vi "FF+FB 適應性控制(系統鑑別).vi"() -> ()   [LabVIEW 2010]
uses:
  <vilib>/DAQmx/read.llb/DAQmx Read (Analog 1D DBL NChan 1Samp).vi
  <vilib>/DAQmx/write.llb/DAQmx Write (Analog DBL 1Chan 1Samp).vi
  <vilib>/DAQmx/create/channels.llb/DAQmx Create Channel (AI-Voltage-Basic).vi
  <vilib>/DAQmx/configure/timing.llb/DAQmx Timing (Sample Clock).vi
  <vilib>/DAQmx/create/channels.llb/DAQmx Create Channel (AO-Voltage-Basic).vi
  <vilib>/daqmx/miscellaneous.llb/DAQmx Fill In Error Info.vi
panel:
  in  "input channels 3":tag="PXI-6229/ai2"
  in  "適應性雜訊消除":bool=TRUE
  in  "u(收斂係數)":dbl=0.02
  in  "order":i32=1000
  in  "ch2-1估測DC時間(秒)":dbl=2.0
  in  "ch2-2 估測DC時間(秒)":dbl=2.0
  in  "ch2 Kii 增益":dbl
  in  "ch2 Kp 增益":dbl=0.13
  out "overload":bool=TRUE
  in  "ch1 Kp 增益":dbl=-23.0
  in  "ch2 Ki 增益":dbl=83.5
  in  "ch1 Ki 增益":dbl=-600.0
  in  "ch1-2估測DC時間(秒)":dbl=2.0
  in  "ch2-3估測DC時間(秒)":dbl=0.1
  in  "Controller on":bool
  out "error out":errorcluster
  out "延遲百分比(%)  需小於0.5%":dbl=0.21369830071382712
  out "理想迴圈時間(ms)":dbl=0.2
  out "迴圈平均運行時間(ms)":dbl=0.20042739660142767
  in  "output channels 1":tag="PXI-6733/ao0"
  in  "stop":bool
  in  "ch1-1估測DC時間(秒)":dbl=2.0
  in  "每通道取樣頻率(Hz)":dbl=5000.0 format="%0.2f"
  in  "input channels 2":tag="PXI-6229/ai1"
  in  "input channels 1":tag="PXI-6229/ai0"
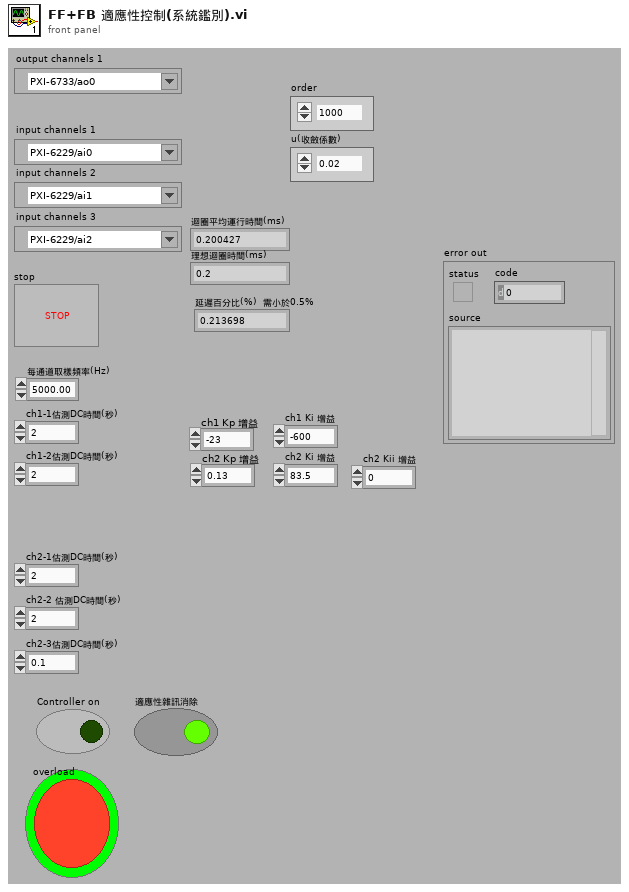
[diagram p1: front panel]
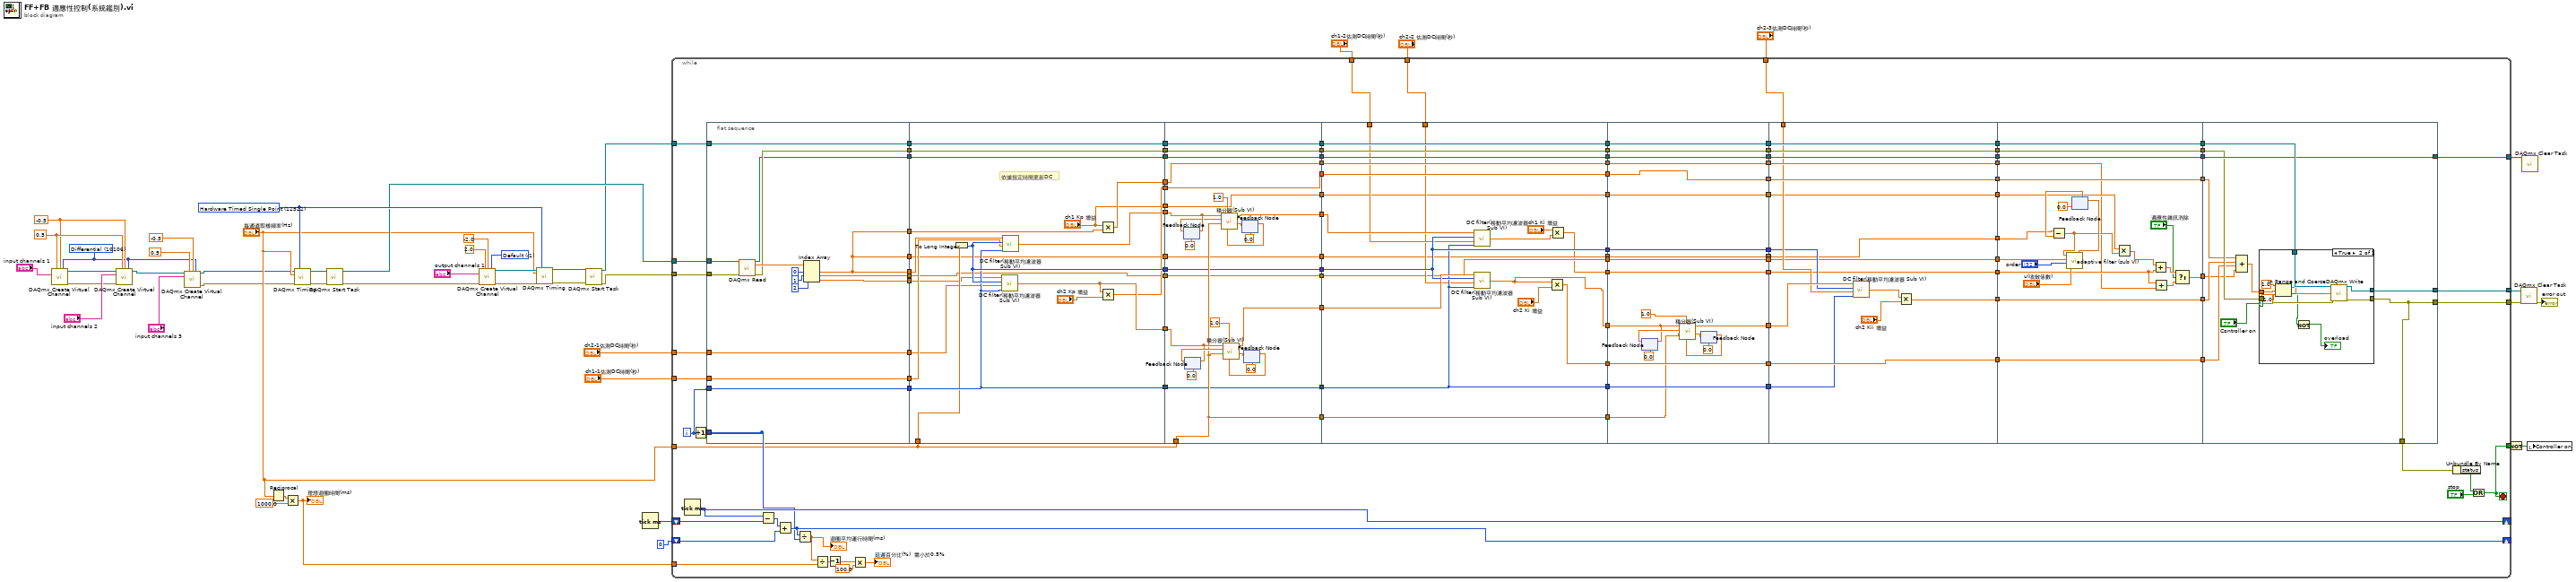
[diagram p0: block diagram]
diagram:
  w35 = -1 items=["Default"=-1, "RSE"=10083, "Differential"=10106, "Pseudodifferential"=12529] ("output terminal configuration")
  w32 = 12522 items=["Finite Samples"=10178, "Continuous Samples"=10123, "Hardware Timed Single Point"=12522] ("sample mode")
  w1 = 10106 items=["default"=-1, "RSE"=10083, "NRSE"=10078, "Differential"=10106, "Pseudodifferential"=12529] ("input terminal configuration")
  w41 = -0.5 ("minimum value")
  w42 = 0.5 ("maximum value")
  n1 = call-poly <vilib>:"DAQmx Create Virtual Channel.vi"("maximum value"=w42, "minimum value"=w41, "input terminal configuration"=w1, "physical channels"="input channels 1") -> ("task out"=w45:refnum<k21>, "error out"=w39:errorcluster)  [unwired: 10 in]
  n2 = call-poly <vilib>:"DAQmx Create Virtual Channel.vi"("task in"=w45, "maximum value"=w42, "minimum value"=w41, "input terminal configuration"=w1, "physical channels"="input channels 2", "error in"=w39) -> ("task out"=w7:refnum<k21>)  [unwired: 8 in, 1 out]
  n3 = call-poly <vilib>:"DAQmx Create Virtual Channel.vi"("task in"=w7, "maximum value"=0.5, "minimum value"=-0.5, "input terminal configuration"=w1, "physical channels"="input channels 3") -> ("task out"=w6:refnum<k21>, "error out"=w5:errorcluster)  [unwired: 9 in]
  n4 = Reciprocal(x="每通道取樣頻率(Hz)") -> (1/x=w23:dbl)
  n5 = Multiply(x=w23, y=1000.0) -> (x*y=w21:dbl)
  "理想迴圈時間(ms)" <- w21
  n6 = call-poly <vilib>:"DAQmx Timing.vi"("task/channels in"=w6, "sample mode"=w32, "rate"="每通道取樣頻率(Hz)", "error in"=w5) -> ("task out"=w40:refnum<k21>, "error out"=w38:errorcluster)  [unwired: 10 in]
  n7 = call <vilib>:"DAQmx Start Task.vi"("task/channels in"=w40, "error in"=w38) -> ("task out"=w28:refnum<k21>, "error out"=w29:errorcluster)  [unwired: 12 in]
  n8 = call-poly <vilib>:"DAQmx Create Virtual Channel.vi"("maximum value"=2.0, "minimum value"=-2.0 ("maximum value"), "output terminal configuration"=w35, "physical channels"="output channels 1", "error in"=w29) -> ("task out"=w34:refnum<k21>, "error out"=w33:errorcluster)  [unwired: 9 in]
  n9 = call-poly <vilib>:"DAQmx Timing.vi"("task/channels in"=w34, "sample mode"=w32, "rate"="每通道取樣頻率(Hz)", "error in"=w33) -> ("task out"=w31:refnum<k21>, "error out"=w30:errorcluster)  [unwired: 10 in]
  n10 = call <vilib>:"DAQmx Start Task.vi"("task/channels in"=w31, "error in"=w30) -> ("task out"=w19:refnum<k21>, "error out"=w27:errorcluster)  [unwired: 12 in]
  n11 = Tick Count (ms)() -> (millisecond timer value=w25:u32)
  n12 = while {
    tunnel: w28 -> [w155]
    tunnel: w27 -> [w154]
    shift-right: [w151] -> _
    shift-left: w25 -> [w152]
    shift-right: [w148] -> _
    shift-left: 0 ("index") -> [w149]
    tunnel: w21 -> [w145]
    tunnel: "每通道取樣頻率(Hz)" -> [w102]
    tunnel: w19 -> [w132]
    tunnel: [w126] -> w16
    tunnel: [w100] -> w15
    tunnel: [w115] -> w14
    tunnel: "ch1-1估測DC時間(秒)" -> [w114]
    tunnel: [w101] -> w12
    tunnel: "ch1-2估測DC時間(秒)" -> [w86]
    tunnel: "ch2-3估測DC時間(秒)" -> [w85]
    tunnel: "ch2-2 估測DC時間(秒)" -> [w84]
    tunnel: "ch2-1估測DC時間(秒)" -> [w83]
    i -> [w112]
    stop <- w101 stop-if-true
    n13 = Tick Count (ms)() -> (millisecond timer value=w151:u32)
    n14 = Increment(x=w112) -> (x+1=w147:i32)
    n15 = flat-sequence {
      tunnel: w155 -> [w170]
      tunnel: w154 -> [w169]
      tunnel: [w158] -> w153
      tunnel: w147 -> [_]
      tunnel: w132 -> [w165]
      tunnel: [w165] -> w127
      tunnel: [w164] -> w125
      tunnel: [w163] -> w120
      tunnel: w114 -> [w162]
      tunnel: [w162] -> w113
      tunnel: w112 -> [w161]
      tunnel: [w161] -> w111
      tunnel: w83 -> [w160]
      tunnel: [w160] -> w82
      tunnel: [w158] -> w63
      tunnel: [w159] -> w62
      tunnel: [w158] -> w53
      tunnel: [w156] -> w46
      tunnel: w153 -> [w186]
      tunnel: [w179] -> w140
      tunnel: [w176] -> w139
      tunnel: [w189] -> w128
      tunnel: w127 -> [w189]
      tunnel: w125 -> [w188]
      tunnel: [w188] -> w124
      tunnel: w120 -> [w187]
      tunnel: [w187] -> w116
      tunnel: w113 -> [w184]
      tunnel: w111 -> [w183]
      tunnel: [w185] -> w109
      tunnel: [w183] -> w107
      tunnel: w102 -> [w182]
      tunnel: [w181] -> w95
      tunnel: [w178] -> w91
      tunnel: w82 -> [w177]
      tunnel: [w175] -> w64
      tunnel: w63 -> [w175]
      tunnel: w62 -> [w174]
      tunnel: [w174] -> w61
      tunnel: w53 -> [w173]
      tunnel: ["ch1 Kp 增益"] -> w48
      tunnel: w46 -> [w171]
      tunnel: w140 -> [w205]
      tunnel: w139 -> [w216]
      tunnel: w102 -> [w202]
      tunnel: [w204] -> w138
      tunnel: [w203] -> w137
      tunnel: [w202] -> w134
      tunnel: [w201] -> w129
      tunnel: w128 -> [w201]
      tunnel: w124 -> [w200]
      tunnel: [w200] -> w122
      tunnel: [w199] -> w117
      tunnel: w116 -> [w199]
      tunnel: [w198] -> w110
      tunnel: w109 -> [w198]
      tunnel: [w197] -> w108
      tunnel: w107 -> [w197]
      tunnel: w95 -> [w194]
      tunnel: [w194] -> w92
      tunnel: w91 -> [w193]
      tunnel: [w193] -> w90
      tunnel: [w192] -> w65
      tunnel: w64 -> [w192]
      tunnel: w61 -> [w191]
      tunnel: [w191] -> w60
      tunnel: [w190] -> w49
      tunnel: w48 -> [w190]
      tunnel: w138 -> [w233]
      tunnel: w137 -> [w232]
      tunnel: [w225] -> w136
      tunnel: [w237] -> w135
      tunnel: w134 -> [w237]
      tunnel: [w236] -> w130
      tunnel: w129 -> [w236]
      tunnel: [w235] -> w123
      tunnel: w122 -> [w235]
      tunnel: [w234] -> w118
      tunnel: w117 -> [w234]
      tunnel: w110 -> [w231]
      tunnel: w108 -> [w230]
      tunnel: [w231] -> w105
      tunnel: [w230] -> w103
      tunnel: [w227] -> w93
      tunnel: w92 -> [w227]
      tunnel: w90 -> [w226]
      tunnel: [w226] -> w88
      tunnel: [w224] -> w87
      tunnel: w86 -> [w223]
      tunnel: w84 -> [w222]
      tunnel: [w221] -> w66
      tunnel: w65 -> [w221]
      tunnel: w60 -> [w220]
      tunnel: [w220] -> w59
      tunnel: [w218] -> w54
      tunnel: [w217] -> w50
      tunnel: w49 -> [w217]
      tunnel: w136 -> [w246]
      tunnel: w135 -> [w242]
      tunnel: [w253] -> w133
      tunnel: [w252] -> w131
      tunnel: w130 -> [w252]
      tunnel: w123 -> [w251]
      tunnel: [w251] -> w121
      tunnel: [w250] -> w119
      tunnel: w118 -> [w250]
      tunnel: [w249] -> w106
      tunnel: w105 -> [w249]
      tunnel: [w248] -> w104
      tunnel: w103 -> [w248]
      tunnel: [w243] -> w96
      tunnel: [w245] -> w94
      tunnel: w93 -> [w245]
      tunnel: [w244] -> w89
      tunnel: w88 -> [w244]
      tunnel: w87 -> [w243]
      tunnel: [w241] -> w67
      tunnel: w66 -> [w241]
      tunnel: w59 -> [w240]
      tunnel: [w240] -> w58
      tunnel: [w239] -> w55
      tunnel: w54 -> [w239]
      tunnel: [w238] -> w51
      tunnel: w50 -> [w238]
      tunnel: w133 -> [w272]
      tunnel: [w275] -> w81
      tunnel: w131 -> [w275]
      tunnel: [w274] -> w79
      tunnel: w121 -> [w274]
      tunnel: [w273] -> w77
      tunnel: w119 -> [w273]
      tunnel: w106 -> [w264]
      tunnel: w104 -> [w266]
      tunnel: [w271] -> w75
      tunnel: w96 -> [w271]
      tunnel: [w270] -> w73
      tunnel: w94 -> [w270]
      tunnel: [w269] -> w72
      tunnel: w89 -> [w269]
      tunnel: [w267] -> w70
      tunnel: w85 -> [w265]
      tunnel: [w262] -> w68
      tunnel: w67 -> [w262]
      tunnel: w58 -> [w261]
      tunnel: [w261] -> w57
      tunnel: [w260] -> w56
      tunnel: w55 -> [w260]
      tunnel: [w259] -> w52
      tunnel: w51 -> [w259]
      tunnel: w81 -> [w297]
      tunnel: [w297] -> w80
      tunnel: w79 -> [w296]
      tunnel: [w296] -> w78
      tunnel: w77 -> [w295]
      tunnel: [w295] -> w76
      tunnel: w75 -> [w294]
      tunnel: [w294] -> w74
      tunnel: w73 -> [w276]
      tunnel: w72 -> [w293]
      tunnel: [w293] -> w71
      tunnel: w70 -> [w290]
      tunnel: [w290] -> w69
      tunnel: w68 -> [w277]
      tunnel: w57 -> [w286]
      tunnel: w56 -> [w283]
      tunnel: w52 -> [w282]
      tunnel: [w278] -> w47
      tunnel: w80 -> [w308]
      tunnel: [w307] -> w126
      tunnel: w78 -> [w304]
      tunnel: [w303] -> w100
      tunnel: [w306] -> w115
      tunnel: w76 -> [w306]
      tunnel: [w303] -> w99
      tunnel: w74 -> [w300]
      tunnel: w71 -> [w302]
      tunnel: w69 -> [w301]
      tunnel: w47 -> [w298]
      frame #0 {
        n16 = call-poly <vilib>:"DAQmx Read.vi"("task/channels in"=w170, "error in"=w169) -> ("task out"=w163:refnum<k21>, "data"=w166:dbl[], "error out"=w164:errorcluster)  [unwired: 11 in]
        n17 = Index Array(array=w166, index #1=0 ("index"), index #2=1 ("index"), index #3=2 ("index")) -> (element #1=w158:dbl, element #2=w159:dbl, element #3=w156:dbl)
      }
      frame #1 {
        # "依據指定時間更新DC"
        n18 = To Long Integer(number=w182) -> (32bit integer=w185:i32)
        n19 = call "DC filter(移動平均濾波器 Sub VI).vi"("當前迴圈計數(i)"=w183, "平均時間"=w177, "取樣頻率(Hz)"=w185, "input signal"=w171) -> ("DC filter output"=w179:dbl)
        n20 = call "DC filter(移動平均濾波器 Sub VI).vi"("當前迴圈計數(i)"=w183, "平均時間"=w184, "取樣頻率(Hz)"=w185, "input signal"=w186) -> ("DC filter output"=w176:dbl)
        n21 = Multiply(x="ch1 Kp 增益", y=w173) -> (x*y=w181:dbl)
        n22 = Multiply(x=w179, y="ch2 Kp 增益") -> (x*y=w178:dbl)
      }
      frame #2 {
        n23 = feedback #1(0.0) -> (w215:dbl)
        n24 = feedback-in #1(w216) -> ()
        n25 = feedback #2(0.0) -> (w206:dbl)
        n26 = feedback-in #2(w205) -> ()
        n27 = feedback #3(0.0 ("輸出累加ERR回朔")) -> (w213:dbl)
        n28 = call "積分器(Sub VI).vi"("輸入累加ERR回朔"=w213, "I增益"=1.0, "samples (Hz)"=w202, "前一個ERR"=w215, "當下ERR"=w216) -> ("輸出累加ERR回朔"=w214:dbl, "積分修正量"=w204:dbl)  [unwired: 5 in]
        n29 = feedback-in #3(w214) -> ()
        n30 = feedback #4(0.0 ("輸出累加ERR回朔")) -> (w208:dbl)
        n31 = call "積分器(Sub VI).vi"("輸入累加ERR回朔"=w208, "I增益"=1.0, "samples (Hz)"=w202, "前一個ERR"=w206, "當下ERR"=w205) -> ("輸出累加ERR回朔"=w207:dbl, "積分修正量"=w203:dbl)  [unwired: 5 in]
        n32 = feedback-in #4(w207) -> ()
      }
      frame #3 {
        n33 = call "DC filter(移動平均濾波器 Sub VI).vi"("當前迴圈計數(i)"=w230, "平均時間"=w223, "取樣頻率(Hz)"=w231, "input signal"=w233) -> ("DC filter output"=w219:dbl)
        n34 = call "DC filter(移動平均濾波器 Sub VI).vi"("當前迴圈計數(i)"=w230, "平均時間"=w222, "取樣頻率(Hz)"=w231, "input signal"=w232) -> ("DC filter output"=w225:dbl)
        n35 = Multiply(x=w225, y="ch2 Ki 增益") -> (x*y=w224:dbl)
        n36 = Multiply(x="ch1 Ki 增益", y=w219) -> (x*y=w218:dbl)
      }
      frame #4 {
        n37 = feedback #5(0.0) -> (w254:dbl)
        n38 = feedback-in #5(w246) -> ()
        n39 = feedback #6(0.0 ("輸出累加ERR回朔")) -> (w256:dbl)
        n40 = call "積分器(Sub VI).vi"("輸入累加ERR回朔"=w256, "I增益"=1.0, "samples (Hz)"=w242, "前一個ERR"=w254, "當下ERR"=w246) -> ("輸出累加ERR回朔"=w255:dbl, "積分修正量"=w253:dbl)  [unwired: 5 in]
        n41 = feedback-in #6(w255) -> ()
      }
      frame #5 {
        n42 = call "DC filter(移動平均濾波器 Sub VI).vi"("當前迴圈計數(i)"=w266, "平均時間"=w265, "取樣頻率(Hz)"=w264, "input signal"=w272) -> ("DC filter output"=w263:dbl)
        n43 = Multiply(x=w263, y="ch2 Kii 增益") -> (x*y=w267:dbl)
      }
      frame #6 {
        n44 = feedback #7(0.0 ("FIR輸出")) -> (w288:dbl)
        n45 = Subtract(x=w277, y=w288) -> (x-y=w284:dbl)
        n46 = call "adaptive filter (sub VI).vi"("u(收斂係數)"="u(收斂係數)", "order"="order", "輸入訊號"=w286, "ERR"=w284) -> ("FIR輸出"=w289:dbl)  [unwired: 1 out]
        n47 = feedback-in #7(w289) -> ()
        n48 = Multiply(x=w282, y=w284) -> (x*y=w285:dbl)
        n49 = Add(x=w285, y=w283) -> (x+y=w281:dbl)
        n50 = Add(x=w283, y=w276) -> (x+y=w280:dbl)
        n51 = Select(t=w281, s="適應性雜訊消除", f=w280) -> (s? t:f=w278:dbl)
      }
      frame #7 {
        n52 = Compound Arithmetic op=ADD(w302, w301, w300, w298) -> (w299:dbl)
        n53 = case shown="True" "Controller on" {
          tunnel: w308 -> [_ w318]
          tunnel: [_ w317] -> w307
          tunnel: w304 -> [_ w316]
          tunnel: [_ w315] -> w303
          tunnel: w299 -> [_ w309]
          frame False {
          }
          frame True {
            n54 = In Range and Coerce(upper limit=1.0, x=w309, lower limit=-1.0) -> (coerced(x)=w314:dbl, In Range?=w311:bool)
            n55 = Not(x=w311) -> (.not. x?=→"overload":bool)
            n56 = call-poly <vilib>:"DAQmx Write.vi"("task/channels in"=w318, "data"=w314, "error in"=w316) -> ("task out"=w317:refnum<k21>, "error out"=w315:errorcluster)  [unwired: 10 in, 1 out]
          }
        }
      }
    }
    n57 = Subtract(x=w151, y=w152) -> (x-y=w150:u32)
    n58 = Add(x=w150, y=w149) -> (x+y=w148:u32)
    n59 = Divide(x=w148, y=w147) -> (x/y=w146:dbl)
    "迴圈平均運行時間(ms)" <- w146
    n60 = Divide(x=w146, y=w145) -> (x/y=w144:dbl)
    n61 = Decrement(x=w144) -> (x-1=w143:dbl)
    n62 = Multiply(x=w143, y=100.0) -> (x*y=→"延遲百分比(%)  需小於0.5%":dbl)
    n63 = Unbundle By Name(w99) -> ("status"=w98:bool)
    n64 = Or(x=w98, y="stop") -> (x .or. y?=w101:bool)
  }
  n65 = Not(x=w12) -> (.not. x?=w13:bool)
  n66 = call <vilib>:"DAQmx Clear Task.vi"("task in"=w16, "error in"=w15) -> ("error out"=→"error out":errorcluster)  [unwired: 13 in]
  n67 = call <vilib>:"DAQmx Clear Task.vi"("task in"=w14) -> ()  [unwired: 14 in, 1 out]
  n68 = local write "Controller on"(w13) -> ()
